vi "RPCVariable.vi"(8 "error in (no error)":errorcluster, 10 "Existing Obj Name":string, 11 "mbed_LVLibrary.lvlib:mbed.lvclass":refnum<class "mbed.lvclass">) -> (0 "error out":errorcluster, 1 "Assigned Name":string, 3 "mbed_LVLibrary.lvlib:ValuePass.lvclass 2":refnum<class "RPCVariable.lvclass">)   [LabVIEW 2011, in "mbed_LVLibrary.lvlib" / "RPCVariable.lvclass"]
uses:
  RPCVariable.lvclass
  Transport Mechanisms/mbed/mbed.lvclass
  <vilib>/Utility/error.llb/DialogType.ctl
  RPCVariable.lvclass/RPCVariable.ctl
panel:
  in  "mbed_LVLibrary.lvlib:ValuePass.lvclass":refnum<class "RPCVariable.lvclass">
  # "Value pass can only connect to existing objects"
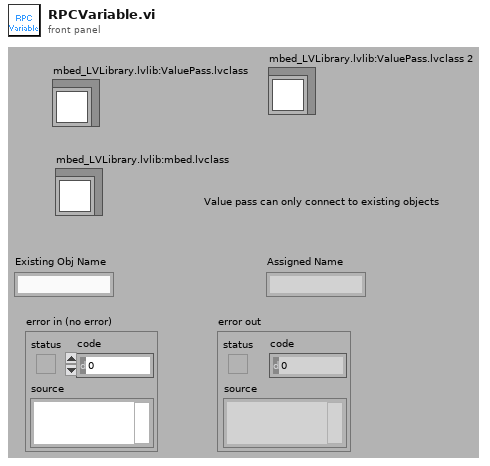
[diagram p1: front panel]
types:
  T1 = typedef "DialogType.ctl" = u16
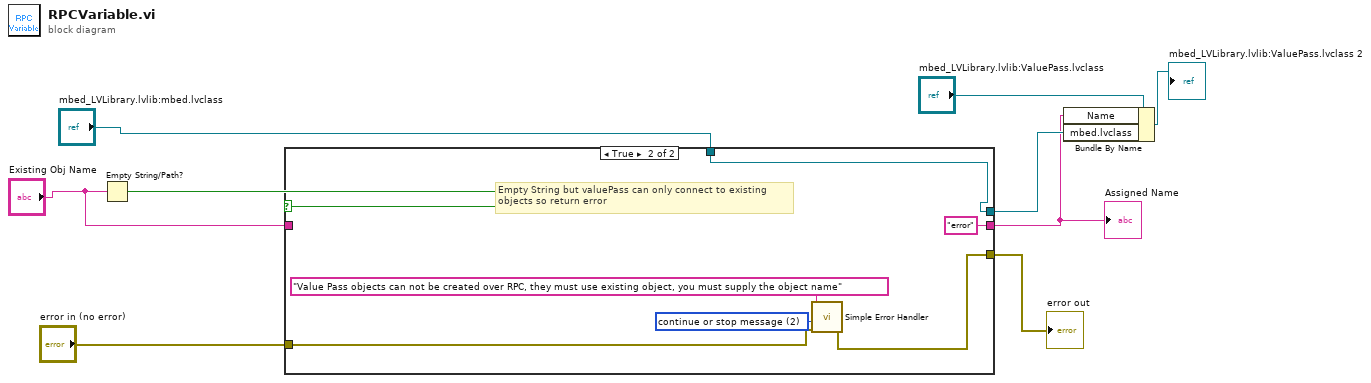
[diagram p0: block diagram]
diagram:
  n1 = Empty String/Path?(string/path="Existing Obj Name") -> (empty?=w6:bool)
  n2 = case shown="True" w6 {
    tunnel: "Existing Obj Name" -> [w12 _]
    tunnel: [w12 "error" ("Existing Obj Name")] -> w7
    tunnel: "mbed_LVLibrary.lvlib:mbed.lvclass" -> [w11 w18]
    tunnel: [w11 w18] -> w8
    tunnel: "error in (no error)" -> [w10 w17]
    tunnel: [w10 w16] -> w4
    frame False {
      # "String present so just set the class name"
    }
    frame True {
      w15 = T1 2 items=["no dialog", "OK message", "continue or stop message", "OK message + warnings", "continue/stop + warnings"] ("type of dialog (OK msg:1)")
      # "Empty String but valuePass can only connect to existing\nobjects so return error"
      n3 = call <vilib>:"Simple Error Handler.vi"("error source (\" \")"="Value Pass objects can not be created over RPC, they must use existing object, you must supply the object name" ("error source (\" \")"), "type of dialog (OK msg:1)"=w15, "error in (no error)"=w17) -> ("error out"=w16:errorcluster)  [unwired: 2 in, 4 out]
    }
  }
  "Assigned Name" <- w7
  "error out" <- w4
  n4 = Bundle By Name(cluster="mbed_LVLibrary.lvlib:ValuePass.lvclass", "Name"=w7, "mbed.lvclass"=w8) -> (→"mbed_LVLibrary.lvlib:ValuePass.lvclass 2":refnum<class "RPCVariable.lvclass">)
